vi "cost.vi"(8 "error in (no error)":errorcluster, 11 "Whip in":refnum<class "Whip.lvclass">) -> (0 "error out":errorcluster, 2 "Cost":dbl, 3 "Whip out":refnum<class "Whip.lvclass">)   [LabVIEW 2013, in "Whip.lvclass"]
uses:
  Whip.lvclass
  Whip.lvclass/Whip.ctl
  Beverage/Beverage.lvclass
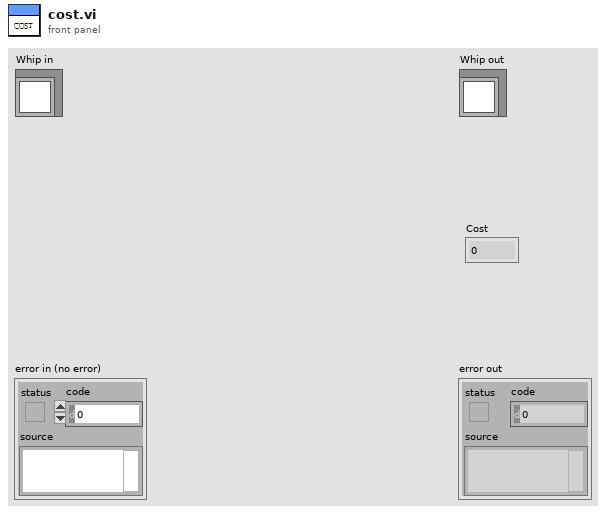
[diagram p1: front panel]
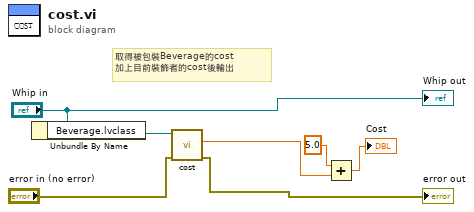
[diagram p0: block diagram]
diagram:
  # "取得被包裝Beverage的cost\n加上目前裝飾者的cost後輸出"
  n1 = Unbundle By Name("Whip in") -> ("Beverage.lvclass"=w5:refnum<class "Beverage.lvclass">)
  n2 = call-dynamic "cost.vi"("error in (no error)"="error in (no error)", "Beverage in"=w5) -> ("error out"=→"error out":errorcluster, "Cost"=w1:dbl)  [unwired: 7 in, 1 out]
  n3 = Add(x=5.0 ("Cost"), y=w1) -> (x+y=→"Cost":dbl)
  "Whip out" <- "Whip in"
